vi "Current Readout.vi"() -> ()   [LabVIEW 2010]
panel:
  out "Current":dbl format="%#.4e"
  in  "Connection On/Off":bool
  in  "Reset on Initialization":bool
  in  "stop":bool
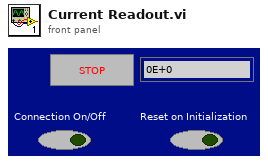
[diagram p1: front panel]
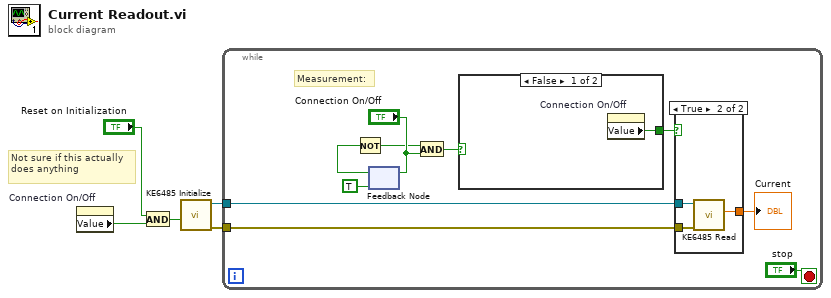
[diagram p0: block diagram]
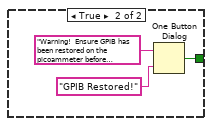
[diagram p2: hidden frame]
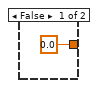
[diagram p3: hidden frame]
diagram:
  # "Not sure if this actually does anything"
  n1 = property on="Connection On/Off" class="Bool (strict)"() -> ("Value"=w2:bool)  [unwired: 2 in, 2 out]
  n2 = And(x="Reset on Initialization", y=w2) -> (x .and. y?=w3:bool)
  n3 = call "KE6485 Initialize.vi"("reset device"=w3) -> ("error out"=w4:errorcluster, "instrument handle out"=w5:refnum<k15>)  [unwired: 9 in]
  n4 = while {
    tunnel: w5 -> [w15]
    tunnel: w4 -> [w14]
    stop <- "stop" stop-if-true
    # "Measurement:"
    n5 = feedback-in #1("Connection On/Off") -> ()
    n6 = feedback #1(TRUE) -> (w11:bool)
    n7 = Not(x=w11) -> (.not. x?=w8:bool)
    n8 = And(x=w8, y="Connection On/Off") -> (x .and. y?=w12:bool)
    n9 = case shown="False" w12 {
      tunnel: [w16 w17] -> w10
      frame False {
        n10 = property on="Connection On/Off" class="Bool (strict)"() -> ("Value"=w16:bool)  [unwired: 2 in, 2 out]
      }
      frame True {
        n11 = One Button Dialog(message="Warning!  Ensure GPIB has been restored on the picoammeter before continuing.  Method to do so:\n1.  Turn on picoammeter\n2.  Press \"Setup\"\n3.  Move down and select \"GPIB\"\n4.  Press \"Enter\"", button name ("OK")="GPIB Restored!") -> (true=w17:bool)
      }
    }
    n12 = case shown="True" w10 {
      tunnel: w15 -> [_ w23]
      tunnel: w14 -> [_ w22]
      tunnel: [0.0 w21] -> w6
      frame False {
      }
      frame True {
        n13 = call "KE6485 Read.vi"("error in (no error)"=w22, "instrument handle"=w23) -> ("reading"=w21:dbl)  [unwired: 7 in, 2 out]
      }
    }
    "Current" <- w6
  }
